vi "Main.vi"() -> ()   [LabVIEW 2020, in "Waters Patrol UPLC Report Parser.lvlib"]
uses:
  Waters Patrol UPLC Report Parser.lvlib
  process loops/Instrument Manager/Instrument State.ctl
  process loops/UI Manager/support/Data Display Loop Data.ctl
  process loops/Logging/Logging Configuration.ctl
  process loops/UI Manager/support/UI Data.ctl
  process loops/UI Manager/support/UI Display State.ctl
  Typedefs/System Control Data.ctl
  <vilib>/Utility/error.llb/Error Cluster From Error Code.vi
  <vilib>/ErrorRing/Error Ring.xnode
  support/Message Queue/Message Queue.lvlib
  support/User Event - Stop/User Event - Stop.lvlib
  process loops/Acquisition/Acquisition.lvlib
  process loops/Instrument Manager/Instrument Manager.lvlib
  process loops/Remote Connection Manager/Remote Connection Manager.lvlib
  process loops/Logging/Logging.lvlib
panel:
  in  "Points to Average":dbl=3.0
  out "Current Data File":path
  in  "Max concentration (mM)":dbl=1.0
  out "Scaled Concentration (mM)":dbl
  out "Peak Data Table":string[][](table)
  in  "Time Interval (sec)":i32=1200
  out "Data Graph":cluster{timestamp[], dbl[]}[](graph)
  in  "Config Log Btn":bool
  in  "Sampling rate\n(sec/sample)":dbl=30.0 min=0.1 step=0.1
  in  "Log Data":bool
  out "Data Directory":path
  # "Waters Patrol Report Parser"
  # "Config"
  # "Peak Data"
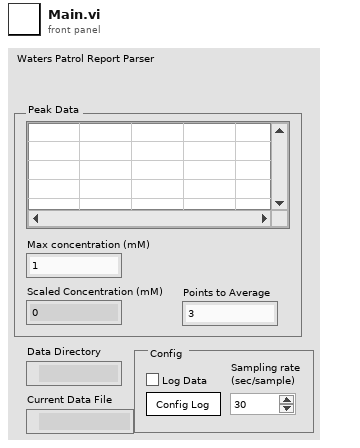
[diagram p1: front panel]
types:
  T1 = typedef "Waters Patrol UPLC Report Parser.lvlib/Data Display Loop Data.ctl" = cluster{"Data Timestamps":timestamp[], "Data Values":dbl[], "Previous Run State":bool}
  T2 = typedef "Waters Patrol UPLC Report Parser.lvlib/Instrument Manager.lvlib/Instrument State.ctl" = cluster{"Data Directory":path, "Last Report Number":i32, "Yield":dbl, "Max Concentration (mM)":dbl, "Report File Pattern":string, "Current Data File":path, "Peak Data Array":cluster{"Time Stamp":timestamp, "Peaks":string[][]}[], "Average Peak Data":cluster{"Time Stamp":timestamp, "Peaks":string[][]}, "Points to Average":i32}
  T3 = typedef "Waters Patrol UPLC Report Parser.lvlib/Message Queue.lvlib/All Message Queues.ctl" = cluster{"System Control":refnum<queue>, "Instrument":refnum<queue>, "Remote":refnum<queue>, "UI":refnum<queue>, "Acquisition":refnum<queue>, "Logging":refnum<queue>}
  T4 = cluster{"Time Stamp":timestamp, "Peaks":string[][]}[]
  T5 = cluster{"Time Stamp":timestamp, "Peaks":string[][]}
  T6 = typedef "Waters Patrol UPLC Report Parser.lvlib/UI Display State.ctl" = enum16{"Shown", "Hidden"}
  T7 = enum8{"Enabled", "Disabled", "Disabled and Grayed Out"}
  T8 = typedef "Waters Patrol UPLC Report Parser.lvlib/UI Data.ctl" = cluster{"Run Btn":refnum<vi>, "Stop Btn":refnum<vi>, "Log Data":refnum<vi>, "Config Log Btn":refnum<vi>, "Sampling rate\n(sec/sample)":refnum<vi>, "Data Graph":refnum<vi>, "Data File Path":refnum<vi>, "Peak Data Table":refnum<vi>, "Yield":refnum<vi>}
  T9 = typedef "Waters Patrol UPLC Report Parser.lvlib/Logging.lvlib/Logging Configuration.ctl" = cluster{"Log Directory Path":path, "Log File Path":path, "Log File Prefix":string, "Log File Extension":string, "File Delimiter":string, "Header Info":string[][], "Channels":string[], "Log Instrument Runs":bool}
  T10 = typedef "Waters Patrol UPLC Report Parser.lvlib/System Control Data.ctl" = cluster{"Log Runs":bool, "Clone":bool}
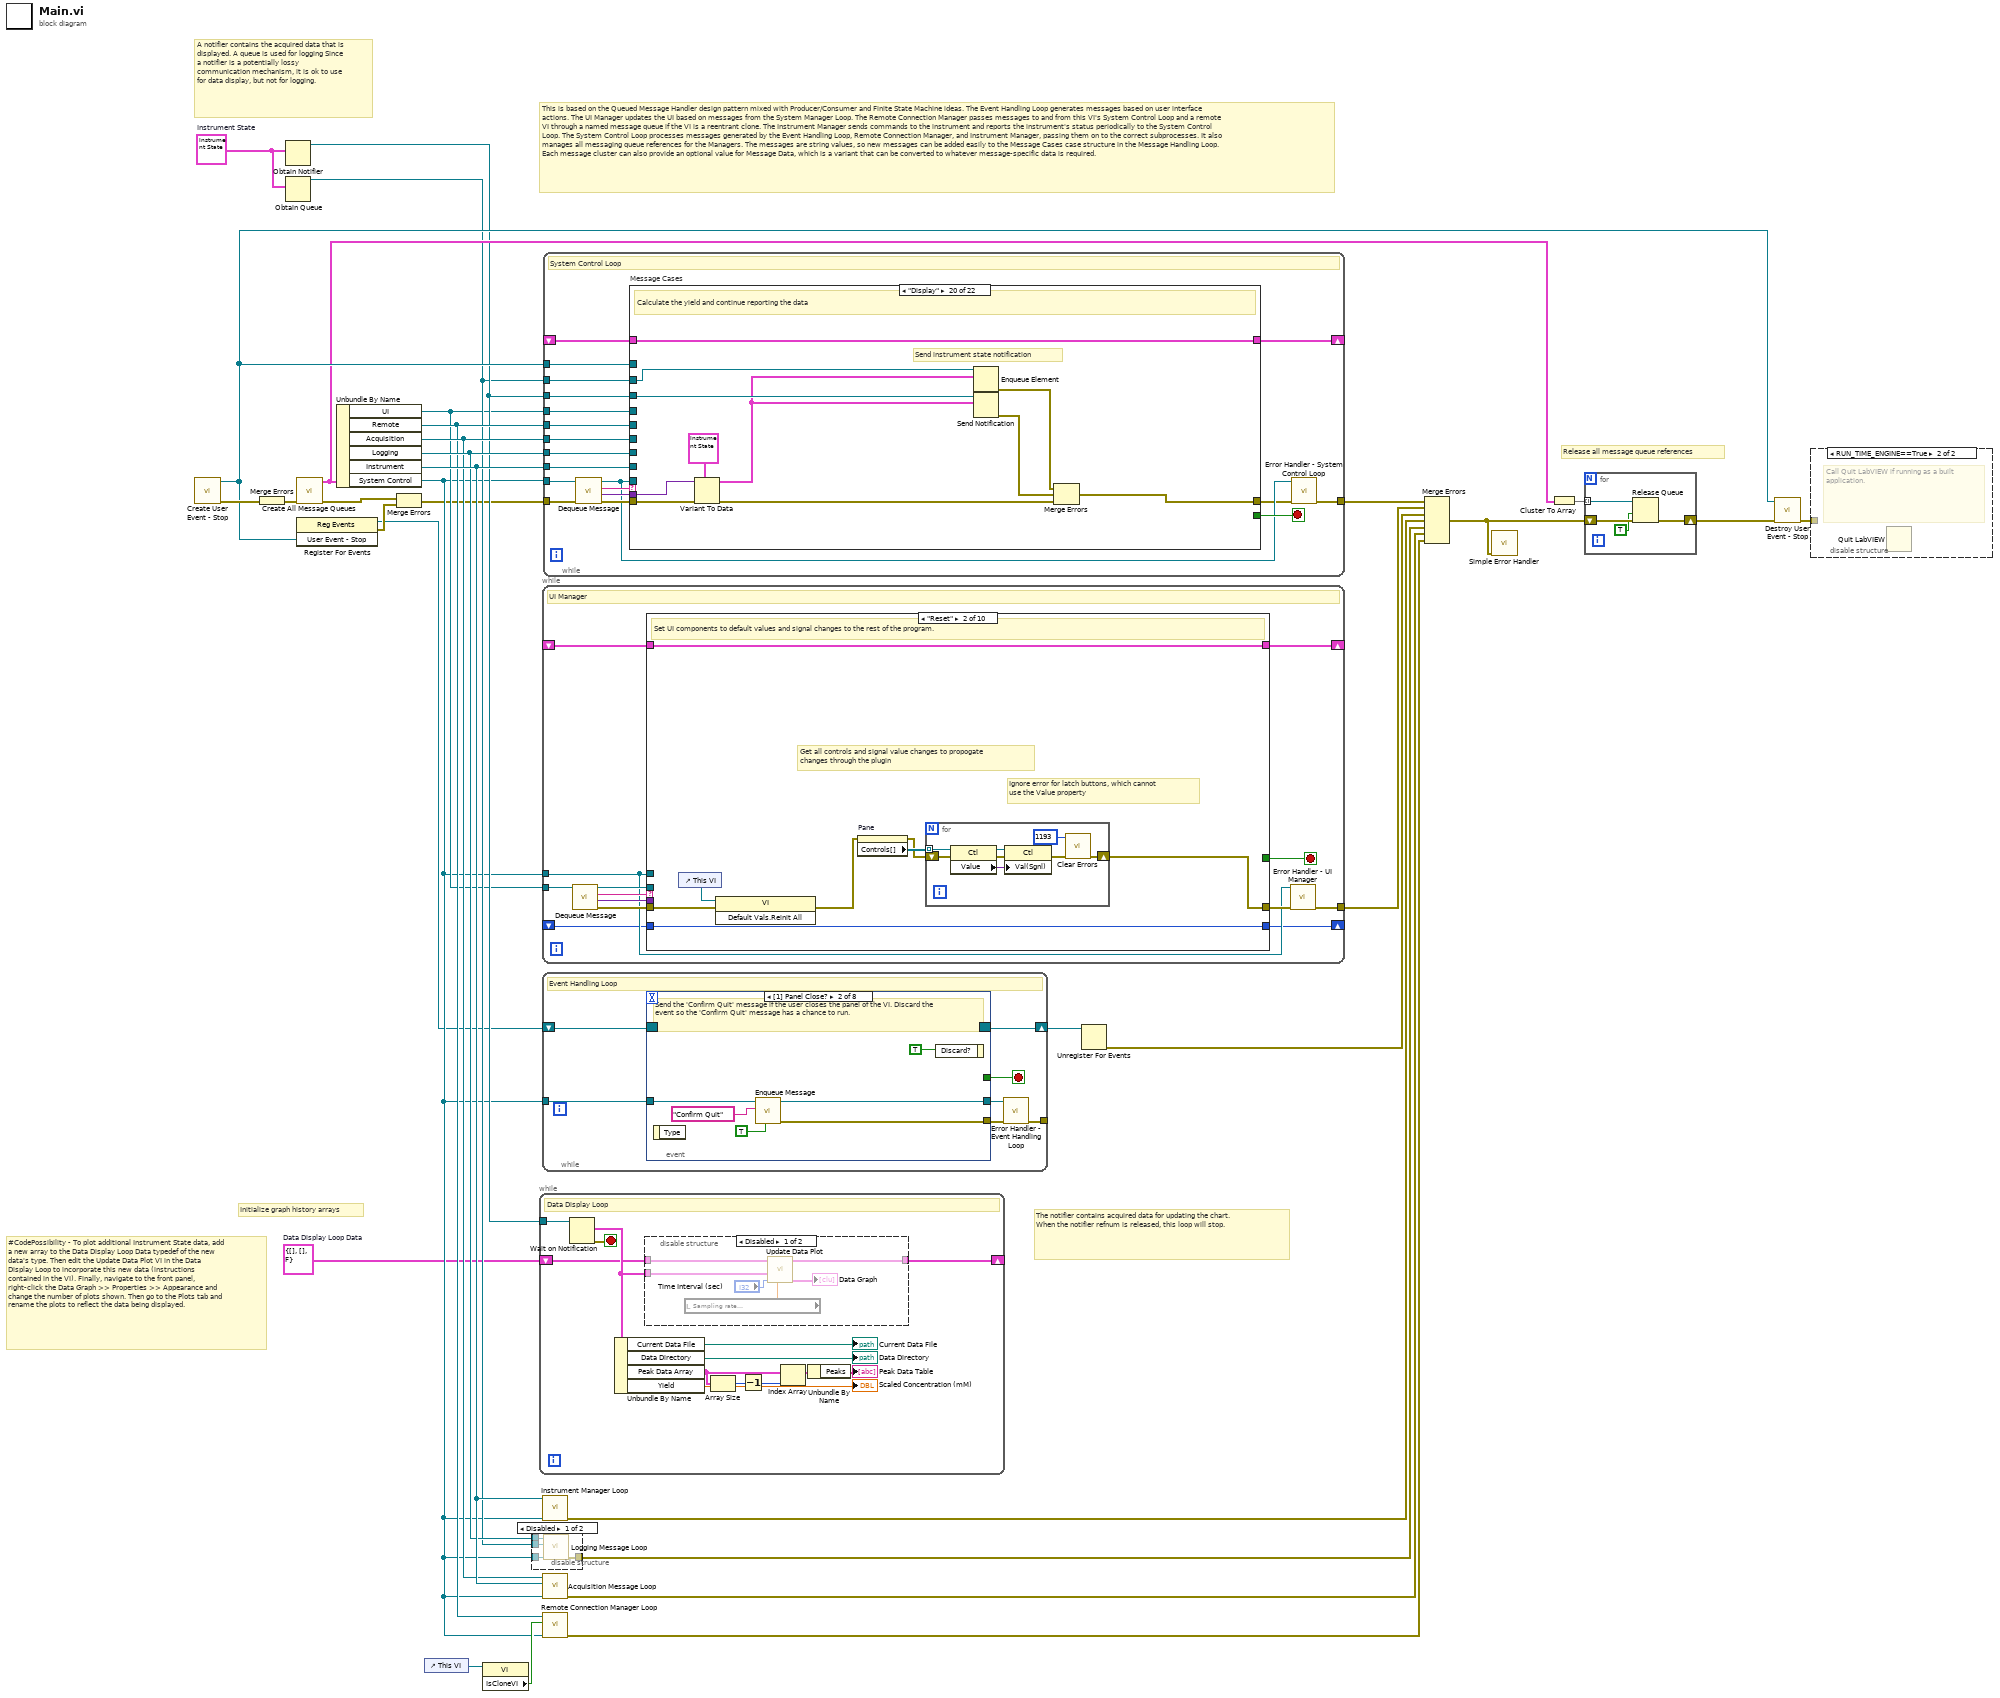
[diagram p0: block diagram]
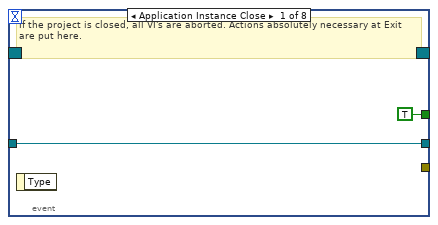
[diagram p4: hidden frame]
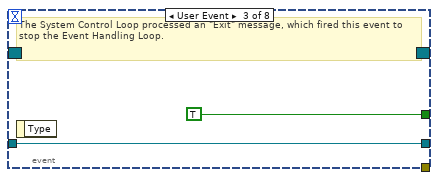
[diagram p5: hidden frame]
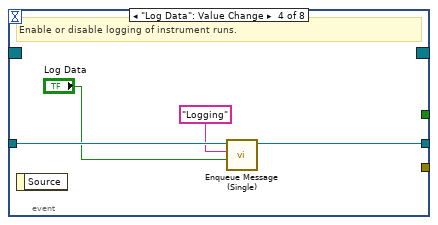
[diagram p6: hidden frame]
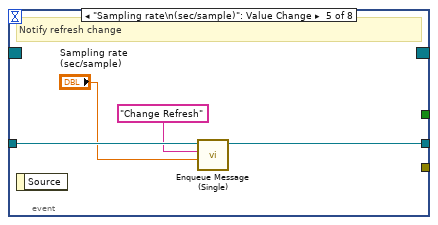
[diagram p7: hidden frame]
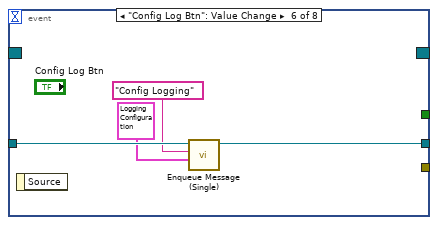
[diagram p8: hidden frame]
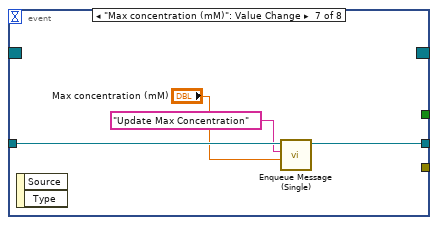
[diagram p9: hidden frame]
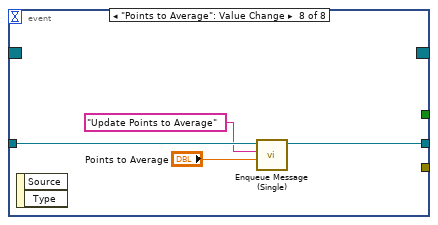
[diagram p10: hidden frame]
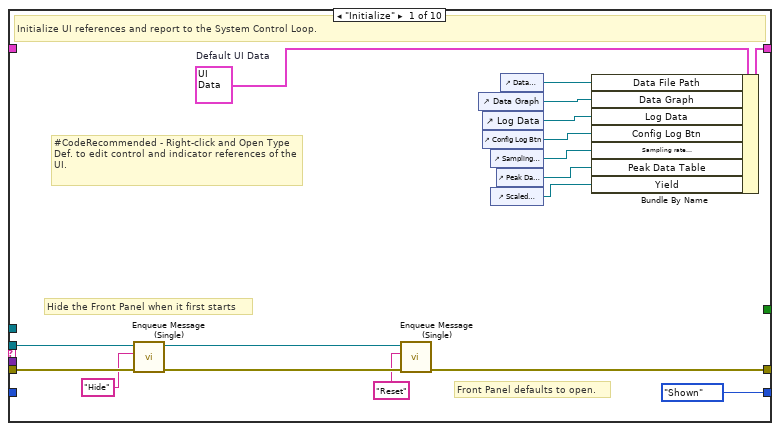
[diagram p11: hidden frame]
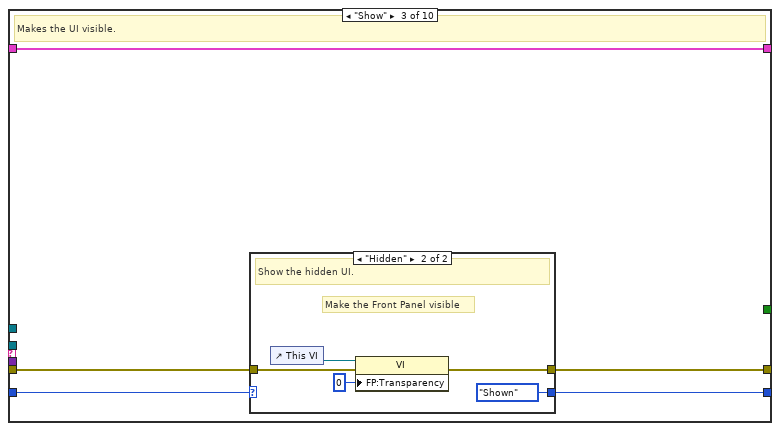
[diagram p12: hidden frame]
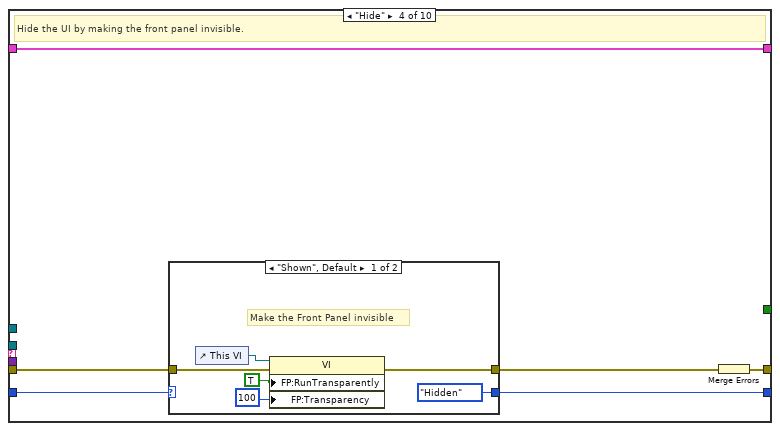
[diagram p14: hidden frame]
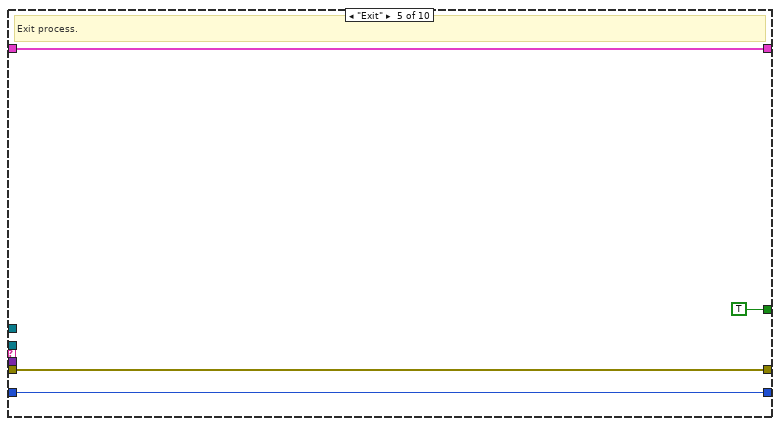
[diagram p16: hidden frame]
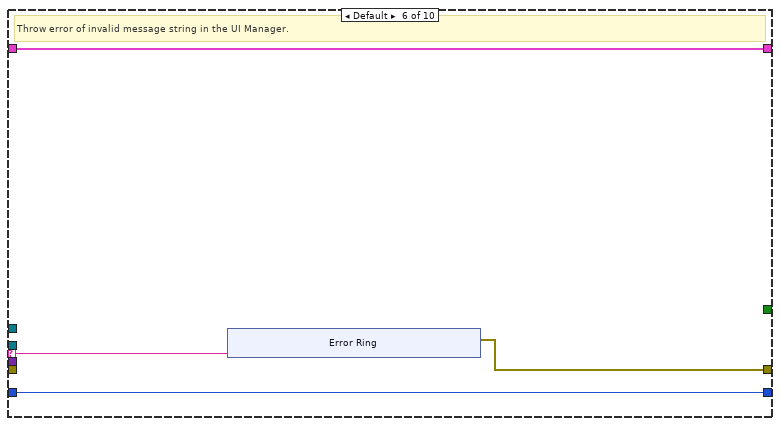
[diagram p17: hidden frame]
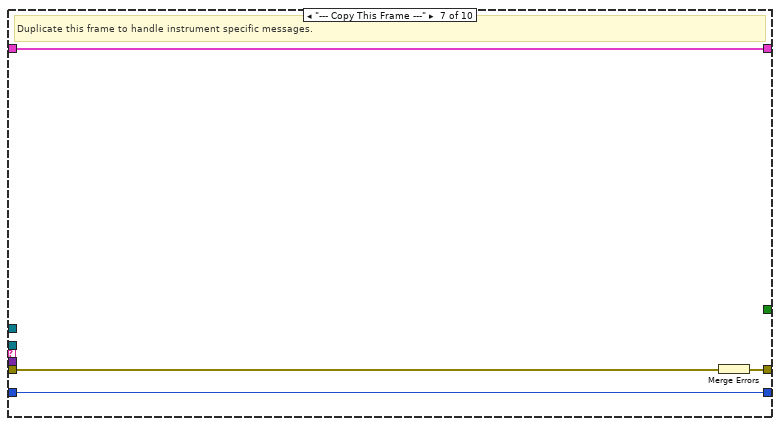
[diagram p18: hidden frame]
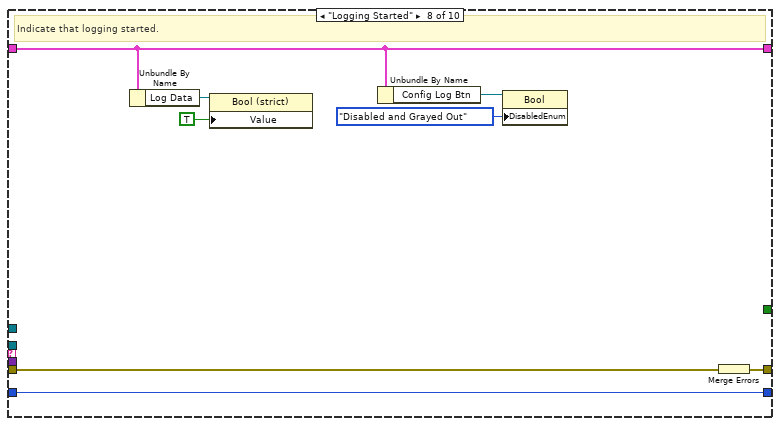
[diagram p19: hidden frame]
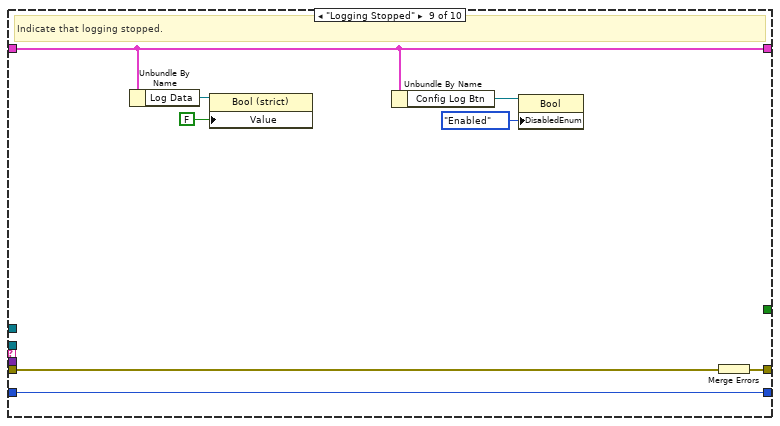
[diagram p20: hidden frame]
diagram:
  w1 = T1 {"Data Timestamps"=[], "Data Values"=[], "Previous Run State"=FALSE}  # Data Display Loop Data
  w7 = T2 {"Data Directory"=path "", "Last Report Number"=0, "Yield"=0.0, "Max Concentration (mM)"=1.0, "Report File Pattern"="", "Current Data File"=path "", "Peak Data Array"=[], "Average Peak Data"={"Time Stamp"=timestamp(0 s since 1904-01-01), "Peaks"=[]}, "Points to Average"=3}  # Instrument State
  # "#CodePossibility - To plot additional Instrument State data, add a new array to the Data Display Loop Data typedef of the new data's type. Then edit the Update Data Plot VI in the Data Display Loop to incorporate this new data (instructions contained in the VI). Finally, navigate to the front panel, right-click the Data Graph >> Properties >> Appearance and change the number of plots shown. Then go to the Plots tab and rename the plots to reflect the data being displayed."
  # "Initialize graph history arrays"
  # "A notifier contains the acquired data that is displayed. A queue is used for logging Since a notifier is a potentially lossy communication mechanism, it is ok to use for data display, but not for logging."
  # "The notifier contains acquired data for updating the chart. When the notifier refnum is released, this loop will stop."
  # "Release all message queue references"
  # "This is based on the Queued Message Handler design pattern mixed with Producer/Consumer and Finite State Machine ideas. The Event Handling Loop generates messages based on user interface actions. The UI Manager updates the UI based on messages from the System Manager Loop. The Remote Connection Manager passes messages to and from this VI's System Control Loop and a remote VI through a named message queue if the VI is a reentrant clone. The Instrument Manager sends commands to the instrument and reports the instrument's status periodically to the System Control Loop. The System Control Loop processes messages generated by the Event Handling Loop, Remote Connection Manager, and Instrument Manager, passing them on to the correct subprocesses. It also manages all messaging queue references for the Managers. The messages are string values, so new messages can be added easily to the Message Cases case structure in the Message Handling Loop.  Each message cluster can also provide an optional value for Message Data, which is a variant that can be converted to whatever message-specific data is required."
  n1 = call "Create User Event - Stop.vi"() -> ("error out"=w26:errorcluster, "User Event - Stop"=w22:refnum<user-event>)  [unwired: 10 in]
  n2 = Merge Errors(w26) -> (w25:errorcluster)
  n3 = Obtain Notifier(notification data type=w7) -> (notifier out=w8:refnum<notifier>)  [unwired: 3 in, 2 out]
  n4 = Obtain Queue(element data type=w7) -> (queue out=w6:refnum<queue>)  [unwired: 4 in, 2 out]
  n5 = call "Create All Message Queues.vi"("error in (no error)"=w25) -> ("error out"=w28:errorcluster, "Message Queues out"=w11:T3)  [unwired: 9 in]
  n6 = register-events(w22) -> (reference out=w2:refnum<event-registration>, error out=w13:errorcluster)  [unwired: 2 in]
  n7 = Unbundle By Name(w11) -> ("UI"=w5:refnum<queue>, "Remote"=w29:refnum<queue>, "Acquisition"=w30:refnum<queue>, "Logging"=w31:refnum<queue>, "Instrument"=w32:refnum<queue>, "System Control"=w4:refnum<queue>)
  n8 = Merge Errors(w28, w13) -> (w3:errorcluster)
  n9 = control-ref of="This VI"() -> (w21:refnum<vi>)
  n10 = property class="VI"(reference=w21) -> ("IsCloneVI"=w20:bool)  [unwired: 1 in, 2 out]
  n11 = disable-structure shown="Disabled" {
    disable-tunnel: w31 -> [w36 _]
    disable-tunnel: [w35 _] -> w16
    disable-tunnel: w6 -> [w34 _]
    disable-tunnel: w4 -> [w33 _]
    frame Disabled {
      n12 = call "Logging Message Loop.vi"("System Control"=w33, "Data Queue"=w34, "Logging"=w36) -> ("error out"=w35:errorcluster)  [unwired: 8 in]
    }
    frame Enabled {
    }
  }
  n13 = while "Data Display Loop" {
    tunnel: w8 -> [w49]
    shift-right: [w44] -> _
    shift-left: w1 -> [w45]
    stop <- w48 stop-if-true
    # "Data Display Loop"
    n14 = Wait on Notification(notifier=w49) -> (notification=w46:T2, error out=w48:errorcluster)  [unwired: 3 in, 2 out]
    n15 = Unbundle By Name(w46) -> ("Current Data File"=→"Current Data File":path, "Data Directory"=→"Data Directory":path, "Peak Data Array"=w39:T4, "Yield"=→"Scaled Concentration (mM)":dbl)
    n16 = disable-structure shown="Disabled" {
      disable-tunnel: w46 -> [w54 _]
      disable-tunnel: w45 -> [w53 _]
      disable-tunnel: [w52 _] -> w44
      frame Disabled {
        n17 = local read "Sampling rate\n(sec/sample)"() -> (w50:dbl)
        n18 = call "Update Data Plot.vi"("Sample Rate (sec/sample)"=w50, "Time interval (s)"="Time Interval (sec)", "Instrument State"=w54, "Graph History Arrays in"=w53) -> ("Updated Graph History"=→"Data Graph":cluster{timestamp[], dbl[]}[], "Graph History Arrays out"=w52:T1)  [unwired: 6 in]
      }
      frame Enabled {
      }
    }
    n19 = Array Size(array=w39) -> (size(s)=w38:i32)
    n20 = Decrement(x=w38) -> (x-1=w37:i32)
    n21 = Index Array(array=w39, index=w37) -> (element=w41:T5)
    n22 = Unbundle By Name(w41) -> ("Peaks"=→"Peak Data Table":string[][])
  }
  n23 = while {
    tunnel: w5 -> [w68]
    tunnel: w4 -> [w59]
    tunnel: [w60] -> w19
    shift-right: [w63] -> _
    shift-left: _ -> [w62]
    shift-right: [w57] -> _
    shift-left: _ -> [w56]
    stop <- w58 stop-if-true
    # "UI Manager"
    n24 = call "Dequeue Message.vi"("Message Queue"=w68) -> ("error out"=w66:errorcluster, "Message Data"=w64:variant, "Message"=w65:string, "dup Message Queue"=w67:refnum<queue>)  [unwired: 7 in]
    n25 = case shown="\"Reset\"" w65 {
      selector: w65 -> [_ _ _ _ _ w135 _ _ _ _]
      tunnel: w67 -> [w81 _ _ _ _ _ _ _ _ _]
      tunnel: w66 -> [w83 w90 w105 w117 w131 _ w144 w153 w161 w169]
      tunnel: w64 -> [_ _ _ _ _ _ _ _ _ w168]
      tunnel: w59 -> [_ _ _ _ _ _ _ _ _ _]
      tunnel: [w71 w86 w104 w118 w131 w134 w145 w154 w162 w170] -> w61
      tunnel: [w84 w91 w106 w119 w130 w133 w146 w149 w155 w164] -> w63
      tunnel: w62 -> [_ w91 w106 w119 w130 w133 w146 w149 w155 w164]
      tunnel: [_ _ _ _ TRUE _ _ _ _ _] -> w58
      tunnel: w56 -> [_ w92 w103 w115 w128 w132 w143 w152 w160 w166]
      tunnel: [UI_Display_State."Shown" ("UI Display State") w92 w102 w114 w128 w132 w143 w152 w160 w166] -> w57
      frame "Initialize" {
        w85 = T8 {"Run Btn"=refnum, "Stop Btn"=refnum, "Log Data"=refnum, "Config Log Btn"=refnum, "Sampling rate\n(sec/sample)"=refnum, "Data Graph"=refnum, "Data File Path"=refnum, "Peak Data Table"=refnum, "Yield"=refnum}  # Default UI Data
        # "Front Panel defaults to open."
        # "Hide the Front Panel when it first starts"
        # "#CodeRecommended - Right-click and Open Type Def. to edit control and indicator references of the UI."
        # "Initialize UI references and report to the System Control Loop."
        n26 = call "Enqueue Message (Single).vi"("error in (no error)"=w83, "Message"="Hide", "Message Queue"=w81) -> ("error out"=w72:errorcluster, "dup Message Queue"=w70:refnum<queue>)  [unwired: 7 in]
        n27 = call "Enqueue Message (Single).vi"("error in (no error)"=w72, "Message"="Reset", "Message Queue"=w70) -> ("error out"=w71:errorcluster)  [unwired: 7 in, 1 out]
        n28 = control-ref of="Data Graph"() -> (w78:refnum<vi>)
        n29 = control-ref of="Log Data"() -> (w77:refnum<vi>)
        n30 = control-ref of="Config Log Btn"() -> (w76:refnum<vi>)
        n31 = control-ref of="Sampling rate (sec/sample)"() -> (w75:refnum<vi>)
        n32 = control-ref of="Scaled Concentration (mM)"() -> (w73:refnum<vi>)
        n33 = control-ref of="Peak Data Table"() -> (w74:refnum<vi>)
        n34 = control-ref of="Data Directory"() -> (w82:refnum<vi>)
        n35 = Bundle By Name(cluster=w85, "Data File Path"=w82, "Data Graph"=w78, "Log Data"=w77, "Config Log Btn"=w76, "Sampling rate\n(sec/sample)"=w75, "Peak Data Table"=w74, "Yield"=w73) -> (w84:T8)
      }
      frame "Reset" {
        # "Ignore error for latch buttons, which cannot\nuse the Value property"
        # "Get all controls and signal value changes to propogate\nchanges through the plugin"
        # "Set UI components to default values and signal changes to the rest of the program."
        n36 = control-ref of="This VI"() -> (w93:refnum<vi>)
        n37 = invoke class="VI" method="Default Vals.Reinit All"(reference=w93, error in=w90) -> (error out=w87:errorcluster)  [unwired: 1 in, 2 out]
        n38 = property on="Pane" class="Pane"(error in=w87) -> (error out=w88:errorcluster, "Controls[]"=w89:refnum<vi>[])  [unwired: 1 in, 1 out]
        n39 = for {
          tunnel: w89 -> [w101] mode=indexing
          shift-right: [w95] -> w86
          shift-left: w88 -> [w100]
          n40 = property class="Ctl"(reference=w101, error in=w100) -> (reference out=w99:refnum<vi>, error out=w98:errorcluster, "Value"=w97:variant)
          n41 = property class="Ctl"(reference=w99, error in=w98, "Val(Sgnl)"=w97) -> (error out=w96:errorcluster)  [unwired: 1 out]
          n42 = call <vilib>:"Clear Errors.vi"("error in (no error)"=w96, "specific error code to clear (0: all)"=1193) -> ("error out"=w95:errorcluster)  [unwired: 4 in, 1 out]
        }
      }
      frame "Show" {
        # "Makes the UI visible."
        n43 = case shown="\"Hidden\"" w103 {
          selector: w103 -> [w108 _]
          tunnel: w105 -> [w107 w113]
          tunnel: [w107 w111] -> w104
          tunnel: [w108 UI_Display_State."Shown" ("UI Display State")] -> w102
          frame "Shown", Default {
            # "Do nothing if UI is already shown."
          }
          frame "Hidden" {
            # "Make the Front Panel visible"
            # "Show the hidden UI."
            n44 = control-ref of="This VI"() -> (w112:refnum<vi>)
            n45 = property class="VI"(reference=w112, error in=w113, "FP:Transparency"=u8 0 ("Front Panel Window:Transparency")) -> (error out=w111:errorcluster)  [unwired: 1 out]
          }
        }
      }
      frame "Hide" {
        # "Hide the UI by making the front panel invisible."
        n46 = case shown="\"Shown\", Default" w115 {
          selector: w115 -> [_ w127]
          tunnel: w117 -> [w122 w126]
          tunnel: [w121 w126] -> w116
          tunnel: [UI_Display_State."Hidden" ("UI Display State") w127] -> w114
          frame "Shown", Default {
            # "Make the Front Panel invisible"
            n47 = control-ref of="This VI"() -> (w125:refnum<vi>)
            n48 = property class="VI"(reference=w125, error in=w122, "FP:RunTransparently"=TRUE ("Front Panel Window:Run VI Transparently"), "FP:Transparency"=u8 100 ("Front Panel Window:Transparency")) -> (error out=w121:errorcluster)  [unwired: 1 out]
          }
          frame "Hidden" {
          }
        }
        n49 = Merge Errors(w116) -> (w118:errorcluster)
      }
      frame "Exit" {
        # "Exit process."
      }
      frame Default {
        # "Throw error of invalid message string in the UI Manager."
        n50 = xnode "Error Ring"("parameter 0"=w135) -> ("error out"=w134:errorcluster)
      }
      frame "--- Copy This Frame ---" {
        # "Duplicate this frame to handle instrument specific messages."
        n51 = Merge Errors(w144) -> (w145:errorcluster)
      }
      frame "Logging Started" {
        # "Indicate that logging started."
        n52 = Unbundle By Name(w149) -> ("Log Data"=w151:refnum<vi>)
        n53 = property class="Bool (strict)"(reference=w151, "Value"=TRUE ("Log Data")) -> ()  [unwired: 1 in, 2 out]
        n54 = Unbundle By Name(w149) -> ("Config Log Btn"=w148:refnum<vi>)
        n55 = property class="Bool"(reference=w148, "DisabledEnum"=T7."Disabled and Grayed Out" ("Disabled")) -> ()  [unwired: 1 in, 2 out]
        n56 = Merge Errors(w153) -> (w154:errorcluster)
      }
      frame "Logging Stopped" {
        # "Indicate that logging stopped."
        n57 = Unbundle By Name(w155) -> ("Log Data"=w159:refnum<vi>)
        n58 = property class="Bool (strict)"(reference=w159, "Value"=FALSE ("Log Data")) -> ()  [unwired: 1 in, 2 out]
        n59 = Unbundle By Name(w155) -> ("Config Log Btn"=w157:refnum<vi>)
        n60 = property class="Bool"(reference=w157, "DisabledEnum"=T7."Enabled" ("Disabled")) -> ()  [unwired: 1 in, 2 out]
        n61 = Merge Errors(w161) -> (w162:errorcluster)
      }
      frame "Change Refresh" {
        # "Update sample rate multiplier in the UI data chart and config indicator."
        n62 = Unbundle By Name(w164) -> ("Sampling rate\n(sec/sample)"=w165:refnum<vi>)
        n63 = Variant To Data(type=0.0, Variant=w168) -> (data=w163:dbl)  [unwired: 1 in, 1 out]
        n64 = property class="DigNum (strict)"(reference=w165, "Value"=w163) -> ()  [unwired: 1 in, 2 out]
        n65 = Merge Errors(w169) -> (w170:errorcluster)
      }
    }
    n66 = call "Error Handler - UI Manager.vi"("error in (no error)"=w61, "Message Queue"=w59) -> ("dup error in"=w60:errorcluster)  [unwired: 8 in, 1 out]
  }
  n67 = while {
    tunnel: w4 -> [w177]
    shift-right: [w175] -> w23
    shift-left: w2 -> [w176]
    tunnel: [w171] -> _
    stop <- w173 stop-if-true
    # "Event Handling Loop"
    n68 = event shown="[1] Panel Close?" {
      selector: w176 -> [_ _ _ _ _ _ _ _]
      dyn-events: [_ _ _ _ _ _ _ _] -> w175
      timeout: _ -> [_ _ _ _ _ _ _ _]
      tunnel: [TRUE ("Discard?") _ TRUE ("Discard?") _ _ _ _ _] -> w173
      tunnel: w177 -> [w179 w184 w187 w191 w195 w199 w203 w207]
      tunnel: [_ w183 _ _ _ _ _ _] -> w174
      tunnel: [w179 w182 w187 w190 w194 w198 w202 w206] -> w172
      event Application Instance Close {
        # "If the project is closed, all VI's are aborted. Actions absolutely necessary at Exit are put here."
        n69 = event-data() -> ()  [unwired: 1 in, 1 out]
      }
      event Panel Close? {
        # "Send the 'Confirm Quit' message if the user closes the panel of the VI. Discard the event so the 'Confirm Quit' message has a chance to run."
        n70 = event-data() -> ()  [unwired: 1 in, 1 out]
        n71 = call-poly "Enqueue Message.vi"("Priority Message? (F)"=TRUE, "Message"="Confirm Quit", "Message Queue"=w184) -> ("error out"=w183:errorcluster, "dup Message Queue"=w182:refnum<queue>)  [unwired: 7 in]
        n72 = event-data("Discard?"=TRUE) -> ()  [unwired: 1 in, 1 out]
      }
      event User Event {
        # "The System Control Loop processed an \"Exit\" message, which fired this event to stop the Event Handling Loop."
        n73 = event-data() -> ()  [unwired: 1 in, 1 out]
      }
      event "Log Data": Value Change {
        # "Enable or disable logging of instrument runs."
        n74 = event-data() -> ()  [unwired: 1 in, 1 out]
        n75 = call "Enqueue Message (Single).vi"("Message Data"="Log Data", "Message"="Logging", "Message Queue"=w191) -> ("dup Message Queue"=w190:refnum<queue>)  [unwired: 7 in, 1 out]
      }
      event "Sampling rate\n(sec/sample)": Value Change {
        # "Notify refresh change"
        n76 = event-data() -> ()  [unwired: 1 in, 1 out]
        n77 = call "Enqueue Message (Single).vi"("Message Data"="Sampling rate\n(sec/sample)", "Message"="Change Refresh", "Message Queue"=w195) -> ("dup Message Queue"=w194:refnum<queue>)  [unwired: 7 in, 1 out]
      }
      event "Config Log Btn": Value Change {
        n78 = event-data() -> ()  [unwired: 1 in, 1 out]
        n79 = call "Enqueue Message (Single).vi"("Message Data"=T9 {"Log Directory Path"=path "", "Log File Path"=path "", "Log File Prefix"="Experiment", "Log File Extension"="csv", "File Delimiter"=",", "Header Info"=[], "Channels"=[], "Log Instrument Runs"=FALSE} ("Logging Configuration"), "Message"="Config Logging", "Message Queue"=w199) -> ("dup Message Queue"=w198:refnum<queue>)  [unwired: 7 in, 1 out]
      }
      event "Max concentration (mM)": Value Change {
        n80 = event-data() -> ()  [unwired: 1 in, 2 out]
        n81 = call "Enqueue Message (Single).vi"("Message Data"="Max concentration (mM)", "Message"="Update Max Concentration", "Message Queue"=w203) -> ("dup Message Queue"=w202:refnum<queue>)  [unwired: 7 in, 1 out]
      }
      event "Points to Average": Value Change {
        n82 = event-data() -> ()  [unwired: 1 in, 2 out]
        n83 = call "Enqueue Message (Single).vi"("Message Data"="Points to Average", "Message"="Update Points to Average", "Message Queue"=w207) -> ("dup Message Queue"=w206:refnum<queue>)  [unwired: 7 in, 1 out]
      }
    }
    n84 = call "Error Handler - Event Handling Loop.vi"("error in (no error)"=w174, "Message Queue"=w172) -> ("dup error in"=w171:errorcluster)  [unwired: 8 in, 1 out]
  }
  n85 = call "Instrument Manager Loop.vi"("System Control"=w4, "Instrument Manager"=w32) -> ("error out"=w17:errorcluster)  [unwired: 9 in]
  n86 = call "Acquisition Message Loop.vi"("System Control"=w4, "Instrument Manager"=w32, "Acquisition"=w30) -> ("error out"=w15:errorcluster)  [unwired: 8 in]
  n87 = call "Remote Connection Manager Loop.vi"("System Control"=w4, "IsCloneVI (false)"=w20, "Remote"=w29) -> ("error out"=w14:errorcluster)  [unwired: 8 in]
  n88 = while {
    tunnel: w4 -> [w218]
    shift-right: [w225] -> _
    shift-left: _ -> [w226]
    tunnel: w22 -> [w223]
    tunnel: w3 -> [w222]
    tunnel: [w216] -> w27
    tunnel: w32 -> [w214]
    tunnel: w29 -> [w213]
    tunnel: w5 -> [w212]
    tunnel: w30 -> [w211]
    tunnel: w31 -> [w210]
    tunnel: w8 -> [w209]
    tunnel: w6 -> [w208]
    stop <- w224 stop-if-true
    # "System Control Loop"
    n89 = call "Dequeue Message.vi"("error in (no error)"=w222, "Message Queue"=w218) -> ("error out"=w221:errorcluster, "Message Data"=w219:variant, "Message"=w220:string, "dup Message Queue"=w217:refnum<queue>)  [unwired: 6 in]
    n90 = case "Message Cases" shown="\"Display\"" w220 {
      selector: w220 -> [_ _ _ w268 w281 w292 w310 w324 w330 _ w376 w383 w390 w397 w404 w414 w428 w443 w467 _ w485 w497]
      tunnel: w217 -> [_ _ w248 _ _ _ _ _ _ _ _ _ _ _ _ _ _ _ _ _ _ _]
      tunnel: w221 -> [w230 w245 w252 _ _ w295 w313 w328 w346 w359 w380 w387 w394 w401 w408 w417 w431 w447 w454 w469 w481 w493]
      tunnel: [w229 w239 w250 w271 w282 w301 w315 w329 w337 w364 w381 w388 w395 w402 w409 w418 w432 w445 w466 w473 w483 w495] -> w215
      tunnel: w226 -> [_ w244 w251 w267 w283 w302 w316 w327 w336 w365 w382 w389 w396 w403 w410 w419 w433 w446 w456 w471 w482 w494]
      tunnel: [w231 w244 w251 w267 w283 w302 w316 w327 w336 w363 w382 w389 w396 w403 w410 w419 w433 w446 w456 w471 w482 w494] -> w225
      tunnel: [_ _ _ TRUE _ _ _ _ _ _ _ _ _ _ _ _ _ _ _ _ _ _] -> w224
      tunnel: w219 -> [_ w243 _ w272 _ w291 w309 w323 w331 w361 w377 w384 w391 w398 w405 w415 w429 w442 w463 w477 w484 w496]
      tunnel: w223 -> [_ _ _ w269 _ _ _ _ _ _ _ _ _ _ _ _ _ _ _ _ _ _]
      tunnel: w214 -> [w228 _ _ w264 _ w296 _ w325 _ _ _ _ _ _ _ _ _ _ _ _ w479 w491]
      tunnel: w213 -> [_ _ _ w263 _ w299 w314 _ w341 _ _ _ _ _ _ w413 w427 _ w465 _ _ _]
      tunnel: w212 -> [_ _ _ w262 _ w298 _ _ w340 _ _ _ _ _ _ w412 w426 w440 _ _ _ _]
      tunnel: w211 -> [_ _ _ w266 _ w300 _ _ w343 _ _ _ _ _ _ _ _ w441 _ _ _ _]
      tunnel: w210 -> [_ _ _ w265 _ w297 _ _ w333 w357 w378 w385 w392 w399 w406 _ _ _ _ _ _ _]
      tunnel: w209 -> [_ _ _ w259 _ _ _ _ _ _ _ _ _ _ _ _ _ _ w464 w478 _ _]
      tunnel: w208 -> [_ _ _ w257 _ _ _ _ _ _ _ _ _ _ _ _ _ _ w460 w474 _ _]
      frame "Initialize" {
        w232 = T10 {"Log Runs"=FALSE, "Clone"=FALSE}  # Default Data
        # "Initialize the system control loop and system."
        n91 = control-ref of="This VI"() -> ()  [unwired: 1 out]
        n92 = property on="Property Node" class="VI"() -> ("IsCloneVI"=w227:bool)  [unwired: 2 in, 2 out]
        n93 = Bundle By Name(cluster=w232, "Clone"=w227) -> (w231:T10)
        n94 = case shown="False" w227 {
          tunnel: w230 -> [w235 w238]
          tunnel: [w234 w238] -> w229
          tunnel: w228 -> [w233 _]
          frame False {
            # "Initiate the VISA Resource selection window if this is not a"
            n95 = call "Enqueue Message (Single).vi"("error in (no error)"=w235, "Message Data"=path "" ("VISA resource out"), "Message"="Set File", "Message Queue"=w233) -> ("error out"=w234:errorcluster)  [unwired: 6 in, 1 out]
          }
          frame True {
            # "Reentrant clone. It is the responsibility of the RCM to send the Set VISA Resource command."
          }
        }
      }
      frame "Error" {
        # "#CodeRecommended - If you ever change the name of this \"Error\" message, you'll need to update the name in the Check Loop Error.vi as well."
        # "#CodeRecommended - Consider creating a system for logging errors in some way. These errors are for notification purposes only. Handling of specific errors should be performed in the message frames that generated the error."
        # "Error - Display an error dialog. This message is sent by the \"Error Handler\" VIs at the end of other loops in this application."
        n96 = Variant To Data(error in=w245, type=errorcluster {"status"=FALSE, "code"=0, "source"=""} ("error constant"), Variant=w243) -> (data=w241:errorcluster, error out=w240:errorcluster)
        n97 = call <vilib>:"Simple Error Handler.vi"("error in (no error)"=w241) -> ()  [unwired: 4 in, 5 out]
        n98 = Merge Errors(w240) -> (w239:errorcluster)
      }
      frame "Confirm Quit" {
        # "Confirm Quit - Message that can confirm whether or not the user wants to exit the application."
        n99 = call-poly "Enqueue Message.vi"("Priority Message? (F)"=TRUE, "error in (no error)"=w252, "Message"="Exit", "Message Queue"=w248) -> ("error out"=w249:errorcluster)  [unwired: 6 in, 1 out]
        n100 = Merge Errors(w249) -> (w250:errorcluster)
      }
      frame "Exit" {
        # "Order other processes to exit"
        # "Begin the application closing procedure by sending \"Exit\" commands to all running processes."
        n101 = Variant To Data(type=errorcluster {"status"=FALSE, "code"=0, "source"=""} ("error constant"), Variant=w272) -> (data=w273:errorcluster)  [unwired: 1 in, 1 out]
        n102 = Build Array(w262, w263, w266, w265, w264) -> (w261:refnum<queue>[])
        n103 = call <vilib>:"Clear Errors.vi"("error in (no error)"=w273, "specific error code to clear (0: all)"=5000) -> ("error out"=w254:errorcluster)  [unwired: 4 in, 1 out]
        n104 = call <vilib>:"Simple Error Handler.vi"("error in (no error)"=w254) -> ()  [unwired: 4 in, 5 out]
        n105 = for {
          tunnel: w268 -> [w279]
          tunnel: w261 -> [w278] mode=indexing
          shift-right: [w277] -> w270
          shift-left: _ -> [w276]
          n106 = call "Enqueue Message (Single).vi"("Priority Message? (F)"=TRUE, "Message"=w279, "Message Queue"=w278) -> ("error out"=w280:errorcluster)  [unwired: 7 in, 1 out]
          n107 = Merge Errors(w280, w276) -> (w277:errorcluster)
        }
        n108 = Release Notifier(notifier=w259) -> (error out=w258:errorcluster)  [unwired: 2 in, 2 out]
        n109 = Release Queue(queue=w257) -> (error out=w255:errorcluster)  [unwired: 2 in, 2 out]
        n110 = call "Fire User Event - Stop.vi"("User Event - Stop"=w269) -> ("error out"=w256:errorcluster)  [unwired: 10 in]
        n111 = Merge Errors(w256, w255, w258, w270) -> (w271:errorcluster)
      }
      frame Default {
        # "'Default' case only runs if there is a message that isn't defined in any of the other cases.  Output a programming error."
        n112 = xnode "Error Ring"("parameter 0"=w281) -> ("error out"=w282:errorcluster)
      }
      frame "---Copy This Frame---" {
        # "Sends the message to each process in the array."
        # "#CodeRecommended - Change connections to build an array of the processes that will receive this message"
        # "Duplicate this frame when creating new messages.  Change this comment in the duplicated frame to describe this message."
        n113 = Build Array(w298, w299, w300, w297, w296) -> (w293:refnum<queue>[])
        n114 = for {
          tunnel: w293 -> [w306] mode=indexing
          tunnel: w292 -> [w308]
          tunnel: w291 -> [w307]
          shift-right: [w305] -> w294
          shift-left: w295 -> [w303]
          n115 = call "Enqueue Message (Single).vi"("Message Data"=w307, "Message"=w308, "Message Queue"=w306) -> ("error out"=w304:errorcluster)  [unwired: 7 in, 1 out]
          n116 = Merge Errors(w304, w303) -> (w305:errorcluster)
        }
        n117 = Merge Errors(w294) -> (w301:errorcluster)
      }
      frame "Set Remote Queue" {
        # "Sends the message to each process in the array."
        # "Bounce this message back to the Remote Control Manager to set the remote queue to publish messages to."
        n118 = Build Array(w314) -> (w311:refnum<queue>[])
        n119 = for {
          tunnel: w311 -> [w320] mode=indexing
          tunnel: w310 -> [w322]
          tunnel: w309 -> [w321]
          shift-right: [w319] -> w312
          shift-left: w313 -> [w317]
          n120 = call "Enqueue Message (Single).vi"("Message Data"=w321, "Message"=w322, "Message Queue"=w320) -> ("error out"=w318:errorcluster)  [unwired: 7 in, 1 out]
          n121 = Merge Errors(w318, w317) -> (w319:errorcluster)
        }
        n122 = Merge Errors(w312) -> (w315:errorcluster)
      }
      frame "Set File" {
        # "Update the data file path."
        n123 = call "Enqueue Message (Single).vi"("error in (no error)"=w328, "Message Data"=w323, "Message"=w324, "Message Queue"=w325) -> ("error out"=w326:errorcluster)  [unwired: 6 in, 1 out]
        n124 = Merge Errors(w326) -> (w329:errorcluster)
      }
      frame "Valid Directory" {
        # "When a valid data directory has been chosen, start the other processes."
        n125 = Unbundle By Name(w336) -> ("Log Runs"=w335:bool)
        n126 = call "Enqueue Message (Single).vi"("error in (no error)"=w346, "Message Data"=w331, "Message"=w330, "Message Queue"=w333) -> ("error out"=w334:errorcluster, "dup Message Queue"=w332:refnum<queue>)  [unwired: 6 in]
        n127 = case shown="True" w335 {
          tunnel: w334 -> [w347 w351]
          tunnel: w332 -> [_ w350]
          tunnel: [w347 w348] -> w344
          frame False {
          }
          frame True {
            n128 = call "Enqueue Message (Single).vi"("error in (no error)"=w351, "Message"="Start", "Message Queue"=w350) -> ("error out"=w348:errorcluster)  [unwired: 7 in, 1 out]
          }
        }
        n129 = call "Enqueue Message (Single).vi"("error in (no error)"=w344, "Message"="Start", "Message Queue"=w343) -> ("error out"=w342:errorcluster)  [unwired: 7 in, 1 out]
        n130 = Unbundle By Name(w336) -> ("Clone"=w338:bool)
        n131 = call "Enqueue Message (Single).vi"("error in (no error)"=w342, "Message Data"=w331, "Message"=w330, "Message Queue"=w341) -> ("error out"=w339:errorcluster)  [unwired: 6 in, 1 out]
        n132 = case shown="False" w338 {
          tunnel: w339 -> [w355 w356]
          tunnel: [w354 w356] -> w337
          tunnel: w340 -> [w353 _]
          frame False {
            # "Show the Front Panel automatically on startup"
            n133 = call "Enqueue Message (Single).vi"("error in (no error)"=w355, "Message"="Show", "Message Queue"=w353) -> ("error out"=w354:errorcluster)  [unwired: 7 in, 1 out]
          }
          frame True {
            # "Reentrant clone. It is the responsibility of the RCM to send \"Show\"."
          }
        }
      }
      frame "Logging" {
        # "Enable or disable logging in the System Data. Run logging is disabled by default."
        n134 = Variant To Data(type=TRUE, Variant=w361) -> (data=w360:bool)  [unwired: 1 in, 1 out]
        n135 = case shown="True" w360 {
          tunnel: w359 -> [w370 w375]
          tunnel: [w369 w374] -> w358
          tunnel: w357 -> [w368 w373]
          frame False {
            n136 = call "Enqueue Message (Single).vi"("Priority Message? (F)"=TRUE, "error in (no error)"=w370, "Message"="Stop", "Message Queue"=w368) -> ("error out"=w369:errorcluster)  [unwired: 6 in, 1 out]
          }
          frame True {
            n137 = call "Enqueue Message (Single).vi"("Priority Message? (F)"=TRUE, "error in (no error)"=w375, "Message"="Start", "Message Queue"=w373) -> ("error out"=w374:errorcluster)  [unwired: 6 in, 1 out]
          }
        }
        n138 = Bundle By Name(cluster=w365, "Log Runs"=w360) -> (w363:T10)
        n139 = Merge Errors(w358) -> (w364:errorcluster)
      }
      frame "Config Logging" {
        # "Pass on Config Logging message to Logging Loop."
        n140 = call "Enqueue Message (Single).vi"("error in (no error)"=w380, "Message Data"=w377, "Message"=w376, "Message Queue"=w378) -> ("error out"=w379:errorcluster)  [unwired: 6 in, 1 out]
        n141 = Merge Errors(w379) -> (w381:errorcluster)
      }
      frame "Set Log Directory" {
        # "Pass on log setting message to Logging Loop."
        n142 = call "Enqueue Message (Single).vi"("error in (no error)"=w387, "Message Data"=w384, "Message"=w383, "Message Queue"=w385) -> ("error out"=w386:errorcluster)  [unwired: 6 in, 1 out]
        n143 = Merge Errors(w386) -> (w388:errorcluster)
      }
      frame "Set Log File Prefix" {
        # "Pass on log setting message to Logging Loop."
        n144 = call "Enqueue Message (Single).vi"("error in (no error)"=w394, "Message Data"=w391, "Message"=w390, "Message Queue"=w392) -> ("error out"=w393:errorcluster)  [unwired: 6 in, 1 out]
        n145 = Merge Errors(w393) -> (w395:errorcluster)
      }
      frame "Set Log File Delimiter" {
        # "Pass on log setting message to Logging Loop."
        n146 = call "Enqueue Message (Single).vi"("error in (no error)"=w401, "Message Data"=w398, "Message"=w397, "Message Queue"=w399) -> ("error out"=w400:errorcluster)  [unwired: 6 in, 1 out]
        n147 = Merge Errors(w400) -> (w402:errorcluster)
      }
      frame "Set Log on Run" {
        # "Pass on log setting message to Logging Loop."
        n148 = call "Enqueue Message (Single).vi"("error in (no error)"=w408, "Message Data"=w405, "Message"=w404, "Message Queue"=w406) -> ("error out"=w407:errorcluster)  [unwired: 6 in, 1 out]
        n149 = Merge Errors(w407) -> (w409:errorcluster)
      }
      frame "Logging Started" {
        # "Pass on Logging Started message to RCM and UI."
        n150 = Build Array(w412, w413) -> (w411:refnum<queue>[])
        n151 = for {
          tunnel: w415 -> [w422]
          tunnel: w414 -> [w421]
          shift-right: [w423] -> w416
          shift-left: w417 -> [w424]
          tunnel: w411 -> [w420] mode=indexing
          n152 = call "Enqueue Message (Single).vi"("error in (no error)"=w424, "Message Data"=w422, "Message"=w421, "Message Queue"=w420) -> ("error out"=w423:errorcluster)  [unwired: 6 in, 1 out]
        }
        n153 = Merge Errors(w416) -> (w418:errorcluster)
      }
      frame "Logging Stopped" {
        # "Pass on Logging Stopped message to RCM and UI."
        n154 = Build Array(w426, w427) -> (w425:refnum<queue>[])
        n155 = for {
          tunnel: w429 -> [w436]
          tunnel: w428 -> [w435]
          shift-right: [w437] -> w430
          shift-left: w431 -> [w438]
          tunnel: w425 -> [w434] mode=indexing
          n156 = call "Enqueue Message (Single).vi"("error in (no error)"=w438, "Message Data"=w436, "Message"=w435, "Message Queue"=w434) -> ("error out"=w437:errorcluster)  [unwired: 6 in, 1 out]
        }
        n157 = Merge Errors(w430) -> (w432:errorcluster)
      }
      frame "Change Refresh" {
        # "#CodeRecommended - If the default refresh time is changed, it must be updated in the UI and Data Acquisition Loop Data typedef."
        # "Change the sampling rate of the instrument. Default is 1 second/sample."
        n158 = Build Array(w440, w441) -> (w439:refnum<queue>[])
        n159 = for {
          tunnel: w443 -> [w450]
          tunnel: w442 -> [w449]
          tunnel: w439 -> [w448] mode=indexing
          shift-right: [w451] -> w444
          shift-left: w447 -> [w452]
          n160 = call "Enqueue Message (Single).vi"("error in (no error)"=w452, "Message Data"=w449, "Message"=w450, "Message Queue"=w448) -> ("error out"=w451:errorcluster)  [unwired: 6 in, 1 out]
        }
        n161 = Merge Errors(w444) -> (w445:errorcluster)
      }
      frame "Report" {
        # "Send instrument state notification"
        # "Notify processes of update"
        # "Calculate the yield and continue reporting the data"
        n162 = Variant To Data(error in=w454, type=T2 {"Data Directory"=path "", "Last Report Number"=0, "Yield"=0.0, "Max Concentration (mM)"=1.0, "Report File Pattern"="", "Current Data File"=path "", "Peak Data Array"=[], "Average Peak Data"={"Time Stamp"=timestamp(0 s since 1904-01-01), "Peaks"=[]}, "Points to Average"=3} ("Instrument State"), Variant=w463) -> (data=w455:T2, error out=w453:errorcluster)
        n163 = Enqueue Element(queue=w460, element=w455) -> (error out=w458:errorcluster)  [unwired: 2 in, 2 out]
        n164 = Send Notification(notification=w455, notifier=w464) -> (error out=w461:errorcluster)  [unwired: 1 in, 1 out]
        n165 = Merge Errors(w458, w461, w453) -> (w459:errorcluster)
        n166 = call "Enqueue Message (Single).vi"("Message Data"=w463, "Message"=w467, "Message Queue"=w465) -> ("error out"=w457:errorcluster)  [unwired: 7 in, 1 out]
        n167 = Merge Errors(w457, w459) -> (w466:errorcluster)
      }
      frame "Display" {
        # "Send instrument state notification"
        # "Calculate the yield and continue reporting the data"
        n168 = Variant To Data(error in=w469, type=T2 {"Data Directory"=path "", "Last Report Number"=0, "Yield"=0.0, "Max Concentration (mM)"=1.0, "Report File Pattern"="", "Current Data File"=path "", "Peak Data Array"=[], "Average Peak Data"={"Time Stamp"=timestamp(0 s since 1904-01-01), "Peaks"=[]}, "Points to Average"=3} ("Instrument State"), Variant=w477) -> (data=w470:T2, error out=w468:errorcluster)
        n169 = Enqueue Element(queue=w474, element=w470) -> (error out=w472:errorcluster)  [unwired: 2 in, 2 out]
        n170 = Send Notification(notification=w470, notifier=w478) -> (error out=w475:errorcluster)  [unwired: 1 in, 1 out]
        n171 = Merge Errors(w472, w475, w468) -> (w473:errorcluster)
      }
      frame "Update Max Concentration" {
        # "Update the recorded stoichiometry."
        n172 = Build Array(w479) -> (w480:refnum<queue>[])
        n173 = for {
          tunnel: w485 -> [w490]
          tunnel: w484 -> [w489]
          shift-right: [w488] -> w483
          shift-left: w481 -> [w487]
          tunnel: w480 -> [w486] mode=indexing
          n174 = call "Enqueue Message (Single).vi"("error in (no error)"=w487, "Message Data"=w489, "Message"=w490, "Message Queue"=w486) -> ("error out"=w488:errorcluster)  [unwired: 6 in, 1 out]
        }
      }
      frame "Update Points to Average" {
        # "Update the number of points to average."
        n175 = Build Array(w491) -> (w492:refnum<queue>[])
        n176 = for {
          tunnel: w497 -> [w502]
          tunnel: w496 -> [w501]
          shift-right: [w500] -> w495
          shift-left: w493 -> [w499]
          tunnel: w492 -> [w498] mode=indexing
          n177 = call "Enqueue Message (Single).vi"("error in (no error)"=w499, "Message Data"=w501, "Message"=w502, "Message Queue"=w498) -> ("error out"=w500:errorcluster)  [unwired: 6 in, 1 out]
        }
      }
    }
    n178 = call "Error Handler - System Control Loop.vi"("error in (no error)"=w215, "Message Queue"=w217) -> ("dup error in"=w216:errorcluster)  [unwired: 8 in, 1 out]
  }
  n179 = Unregister For Events(event registration refnum=w23) -> (error out=w18:errorcluster)  [unwired: 1 in]
  n180 = Merge Errors(w27, w19, w18, w17, w16, w15, w14) -> (w12:errorcluster)
  n181 = call <vilib>:"Simple Error Handler.vi"("error in (no error)"=w12) -> ()  [unwired: 4 in, 5 out]
  n182 = Cluster To Array(cluster=w11) -> (array=w10:refnum<queue>[])
  n183 = for {
    shift-right: [w504] -> w9
    shift-left: w12 -> [w505]
    tunnel: w10 -> [w506] mode=indexing
    n184 = Release Queue(queue=w506, force destroy? (F)=TRUE, error in (no error)=w505) -> (error out=w504:errorcluster)  [unwired: 2 out]
  }
  n185 = call "Destroy User Event - Stop.vi"("error in (no error)"=w9, "User Event - Stop"=w22) -> ("error out"=w24:errorcluster)  [unwired: 9 in]
  n186 = disable-structure shown="RUN_TIME_ENGINE==True" {
    disable-tunnel: w24 -> [_ _]
    frame condition #0 (active) {
    }
    frame condition #1 {
      # "Call Quit LabVIEW if running as a built application."
      n187 = Quit LabVIEW() -> ()  [unwired: 1 in]
    }
  }
